vi "BRig_dataExp_I_anySelect_prev.vi"() -> (2 "output_I_anySelect_prev":i32)   [LabVIEW 2014]
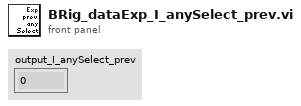
[diagram p1: front panel]
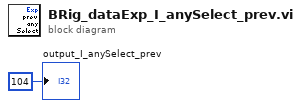
[diagram p0: block diagram]
diagram:
  "output_I_anySelect_prev" <- 104 ("output_iBlock")
